vi "ficheros_subvi.vi"(2 "error in (no error)":errorcluster, 3 "Formato":string, 4 "Nombre del Archivo":string, 5 "Ruta de Almacenamiento":path) -> (0 "error out":errorcluster, 1 "Byte Stream File out":refnum<file>)   [LabVIEW 2020]
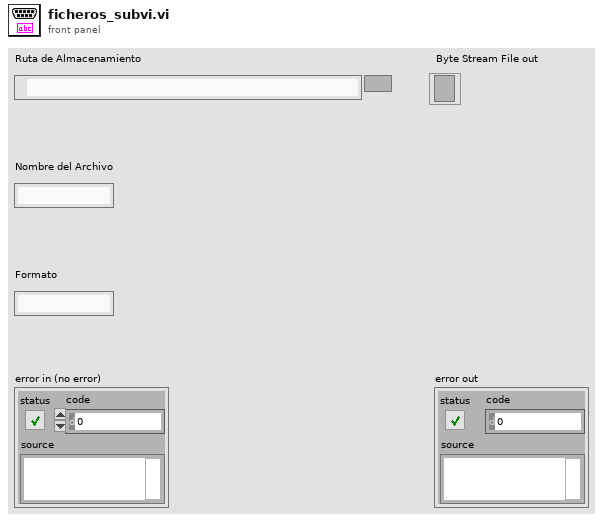
[diagram p1: front panel]
types:
  T1 = enum16{"open", "replace", "create", "open or create", "replace or create", "replace or create with confirmation"}
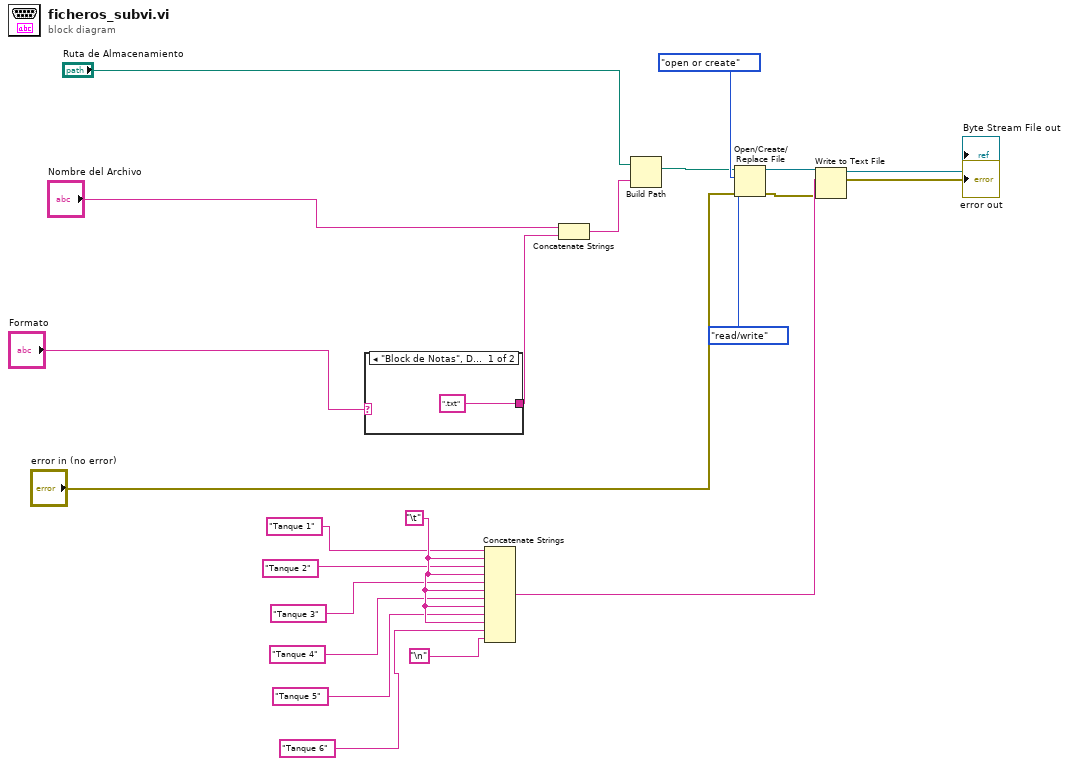
[diagram p0: block diagram]
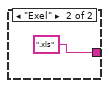
[diagram p2: hidden frame]
diagram:
  w20 = "\t"
  n1 = case shown="\"Block de Notas\", Default" "Formato" {
    tunnel: [".txt" ".xls"] -> w5
    frame "Block de Notas", Default {
    }
    frame "Exel" {
    }
  }
  n2 = Concatenate Strings("Tanque 1", w20, "Tanque 2", w20, "Tanque 3", w20, "Tanque 4", w20, "Tanque 5", w20, "Tanque 6", "\n") -> (w22:string)
  n3 = Concatenate Strings("Nombre del Archivo", w5) -> (w2:string)
  n4 = Build Path(base path="Ruta de Almacenamiento", name or relative path=w2) -> (appended path=w6:path)
  n5 = Open/Create/Replace File(file path (use dialog)=w6, error in="error in (no error)", operation (0:open)=T1."open or create", access (0:read/write)=enum16{"read/write", "read-only", "write-only"}."read/write") -> (refnum out=w10:refnum<file>, error out=w13:errorcluster)  [unwired: 2 in, 1 out]
  n6 = Write to Text File(file (use dialog)=w10, text=w22, error in=w13) -> (refnum out=→"Byte Stream File out":refnum<file>, error out=→"error out":errorcluster)  [unwired: 1 in, 1 out]
